vi "公式复合写入.vi"(11 "公式":cluster{"X^2":dbl, "X":dbl, "b":dbl}) -> ()   [LabVIEW 2016, in "斯坦道总磷.lvlib"]
uses:
  <vilib>/Utility/miscctls.llb/LVPointTypeDef.ctl
panel:
  out "连接的字符串":string
  in  "参数下拉列表":enum16{"总磷", "总氮"}(ring)
  in  "量程下拉列表":enum16{"低量程", "高量程"}(ring)
  in  "取消":bool
  in  "确认":bool
  in  "加标回收":bool
  in  "标样核查":bool
  in  "跨度核查":bool
  in  "空白核查":bool
  in  "水样测量":bool=TRUE
  # "请选择要写入的参数"
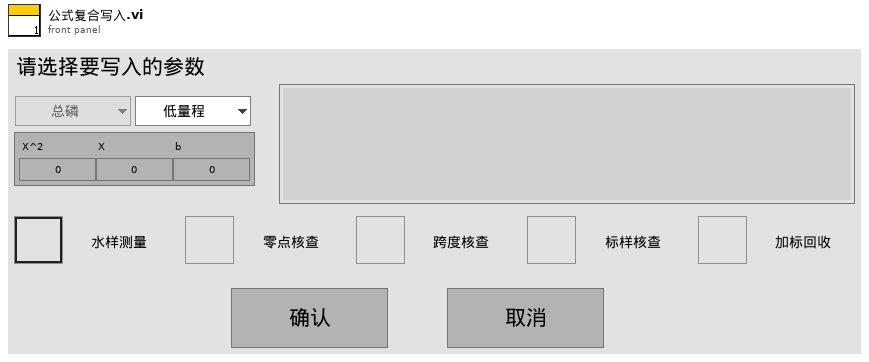
[diagram p1: front panel]
types:
  T1 = typedef "LVPointTypeDef.ctl" = cluster{"Horizontal":i16, "Vertical":i16}
  T2 = cluster{"测量量程":dbl, "测量精度":dbl, "测量间隔":dbl, "消解温度":dbl, "消解时长":dbl, "空白校准时间":timestamp, "曲线截距":dbl, "曲线斜率":dbl, "测量检出限":dbl, "测量信号值":dbl, "线性相关系数":dbl, "二次多项式系数":dbl, "标样校准时间":timestamp, "稀释倍数":dbl, "三项式系数":dbl, "空白标定系数":dbl, "量程系数":dbl, "F0/ORPA":dbl, "F1/ORPB":dbl, "F2/ORPK":dbl, "F3":dbl, "F4":dbl, "F5":dbl, "F6":dbl, "F7":dbl, "X0/滴定数":dbl, "量程":dbl}
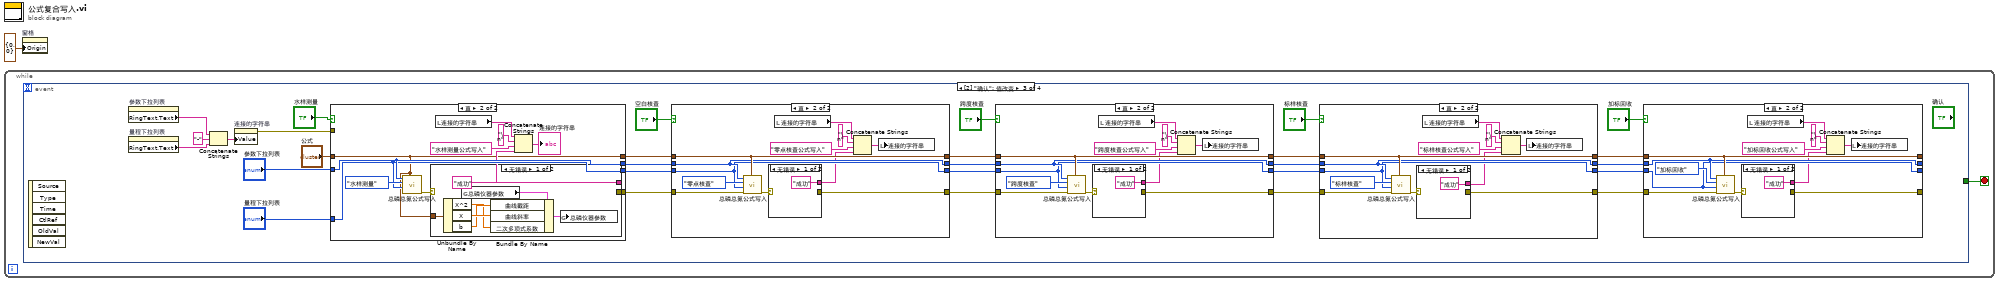
[diagram p0: block diagram]
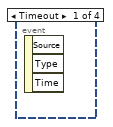
[diagram p2: hidden frame]
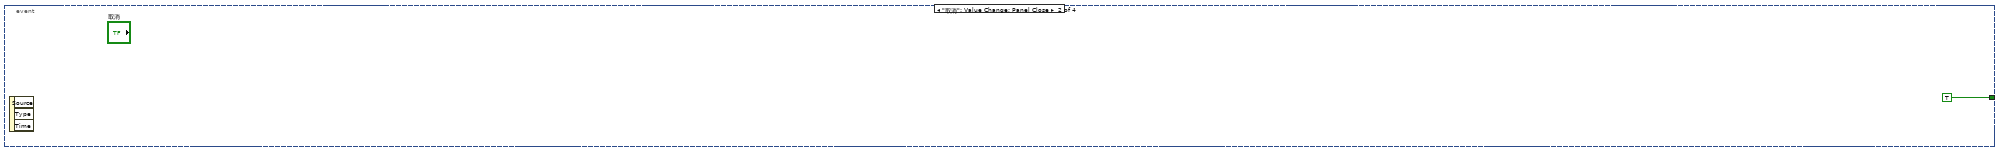
[diagram p3: hidden frame]
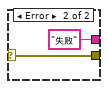
[diagram p5: hidden frame]
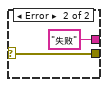
[diagram p7: hidden frame]
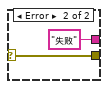
[diagram p9: hidden frame]
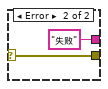
[diagram p11: hidden frame]
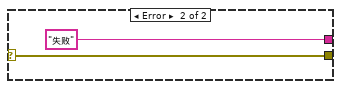
[diagram p13: hidden frame]
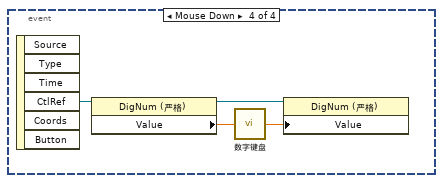
[diagram p14: hidden frame]
diagram:
  n1 = while {
    stop <- w2 stop-if-true
    n2 = event shown="[2] \"确认\": 值改变" {
      selector: _ -> [_ _ _ _]
      dyn-events: _ -> [_ _ _ _]
      timeout: _ -> [_ _ _ _]
      tunnel: [_ TRUE _ _] -> w2
      event Timeout {
        n3 = event-data() -> ()  [unwired: 1 in, 3 out]
      }
      event "取消": Value Change; Panel Close {
        n4 = event-data() -> ()  [unwired: 1 in, 3 out]
      }
      event "确认": Value Change {
        n5 = event-data() -> ()  [unwired: 1 in, 6 out]
        n6 = property on="参数下拉列表" class="Enum (严格)"() -> ("RingText.Text"=w6:string)  [unwired: 2 in, 2 out]
        n7 = property on="量程下拉列表" class="Enum (严格)"() -> ("RingText.Text"=w5:string)  [unwired: 2 in, 2 out]
        n8 = Concatenate Strings(w6, "-" ("字符串"), w5) -> (w7:string)
        n9 = property on="连接的字符串" class="Str"("Value"=w7) -> (error out=w8:errorcluster)  [unwired: 2 in, 1 out]
        n10 = case shown="真" "水样测量" {
          tunnel: "公式" -> [w107 w108]
          tunnel: "参数下拉列表" -> [w106 w117]
          tunnel: "量程下拉列表" -> [w105 w116]
          tunnel: [w107 w108] -> w28
          tunnel: [w106 w117] -> w27
          tunnel: [w105 w116] -> w26
          tunnel: [_ w114] -> w10
          tunnel: w8 -> [_ _]
          frame False {
          }
          frame True {
            n11 = call "总磷总氮公式写入.vi"("公式"=w108, "量程"=w116, "测量模式"=enum16{"水样测量", "零点核查", "跨度核查", "标样核查", "加标回收"}."水样测量", "测量参数"=w117) -> ("error out"=w115:errorcluster)  [unwired: 7 in]
            n12 = case shown="无错误" w115 {
              selector: w115 -> [_ w127]
              tunnel: [_ w127] -> w114
              tunnel: ["成功" "失败"] -> w113
              tunnel: w108 -> [w119 _]
              frame No Error {
                n13 = Unbundle By Name(w119) -> ("X^2"=w122:dbl, "X"=w124:dbl, "b"=w123:dbl)
                n14 = global read "总磷断电保存全局变量.vi" "总磷仪器参数"() -> (w121:T2)
                n15 = Bundle By Name(cluster=w121, "曲线截距"=w123, "曲线斜率"=w124, "二次多项式系数"=w122) -> (w120:T2)
                n16 = global write "总磷断电保存全局变量.vi" "总磷仪器参数"(w120) -> ()
              }
              frame Error {
              }
            }
            n17 = local read "连接的字符串"() -> (w110:string)
            n18 = Concatenate Strings(w110, "\n" ("字符串"), "水样测量公式写入", w113) -> (→"连接的字符串":string)
          }
        }
        n19 = case shown="真" "空白核查" {
          tunnel: w28 -> [w89 w100]
          tunnel: w27 -> [w88 w99]
          tunnel: w26 -> [w87 w98]
          tunnel: [_ w93] -> w25
          tunnel: [w89 w100] -> w24
          tunnel: [w88 w99] -> w23
          tunnel: [w87 w98] -> w22
          tunnel: w10 -> [_ w97]
          frame False {
          }
          frame True {
            n20 = call "总磷总氮公式写入.vi"("公式"=w100, "error in (no error)"=w97, "量程"=w98, "测量模式"=enum16{"水样测量", "零点核查", "跨度核查", "标样核查", "加标回收"}."零点核查", "测量参数"=w99) -> ("error out"=w94:errorcluster)  [unwired: 6 in]
            n21 = case shown="无错误" w94 {
              selector: w94 -> [_ w104]
              tunnel: [_ w104] -> w93
              tunnel: ["成功" "失败"] -> w95
              frame No Error {
              }
              frame Error {
              }
            }
            n22 = local read "连接的字符串"() -> (w92:string)
            n23 = Concatenate Strings(w92, "\n" ("字符串"), "零点核查公式写入", w95) -> (w90:string)
            n24 = local write "连接的字符串"(w90) -> ()
          }
        }
        n25 = case shown="真" "跨度核查" {
          tunnel: w24 -> [w71 w82]
          tunnel: w23 -> [w70 w81]
          tunnel: w22 -> [w69 w80]
          tunnel: [w71 w82] -> w21
          tunnel: [w70 w81] -> w19
          tunnel: [w69 w80] -> w18
          tunnel: w25 -> [_ w79]
          tunnel: [_ w72] -> w9
          frame False {
          }
          frame True {
            n26 = call "总磷总氮公式写入.vi"("公式"=w82, "error in (no error)"=w79, "量程"=w80, "测量模式"=enum16{"水样测量", "零点核查", "跨度核查", "标样核查", "加标回收"}."跨度核查", "测量参数"=w81) -> ("error out"=w73:errorcluster)  [unwired: 6 in]
            n27 = case shown="无错误" w73 {
              selector: w73 -> [_ w86]
              tunnel: [_ w86] -> w72
              tunnel: ["成功" "失败"] -> w74
              frame No Error {
              }
              frame Error {
              }
            }
            n28 = local read "连接的字符串"() -> (w76:string)
            n29 = Concatenate Strings(w76, "\n" ("字符串"), "跨度核查公式写入", w74) -> (w78:string)
            n30 = local write "连接的字符串"(w78) -> ()
          }
        }
        n31 = case shown="真" "标样核查" {
          tunnel: w21 -> [w53 w64]
          tunnel: w19 -> [w52 w63]
          tunnel: w18 -> [w51 w62]
          tunnel: [_ w54] -> w15
          tunnel: [w53 w64] -> w20
          tunnel: [w52 w63] -> w17
          tunnel: [w51 w62] -> w16
          tunnel: w9 -> [_ w61]
          frame False {
          }
          frame True {
            n32 = call "总磷总氮公式写入.vi"("公式"=w64, "error in (no error)"=w61, "量程"=w62, "测量模式"=enum16{"水样测量", "零点核查", "跨度核查", "标样核查", "加标回收"}."标样核查", "测量参数"=w63) -> ("error out"=w55:errorcluster)  [unwired: 6 in]
            n33 = case shown="无错误" w55 {
              selector: w55 -> [_ w68]
              tunnel: [_ w68] -> w54
              tunnel: ["成功" "失败"] -> w56
              frame No Error {
              }
              frame Error {
              }
            }
            n34 = local read "连接的字符串"() -> (w58:string)
            n35 = Concatenate Strings(w58, "\n" ("字符串"), "标样核查公式写入", w56) -> (w60:string)
            n36 = local write "连接的字符串"(w60) -> ()
          }
        }
        n37 = case shown="真" "加标回收" {
          tunnel: w20 -> [w35 w46]
          tunnel: w17 -> [w34 w45]
          tunnel: w16 -> [w33 w44]
          tunnel: [w35 w46] -> _
          tunnel: [w34 w45] -> _
          tunnel: [w33 w44] -> _
          tunnel: w15 -> [_ w43]
          tunnel: [_ w36] -> _
          frame False {
          }
          frame True {
            n38 = call "总磷总氮公式写入.vi"("公式"=w46, "error in (no error)"=w43, "量程"=w44, "测量模式"=enum16{"水样测量", "零点核查", "跨度核查", "标样核查", "加标回收"}."加标回收", "测量参数"=w45) -> ("error out"=w37:errorcluster)  [unwired: 6 in]
            n39 = case shown="无错误" w37 {
              selector: w37 -> [_ w50]
              tunnel: [_ w50] -> w36
              tunnel: ["成功" "失败"] -> w38
              frame No Error {
              }
              frame Error {
              }
            }
            n40 = local read "连接的字符串"() -> (w40:string)
            n41 = Concatenate Strings(w40, "\n" ("字符串"), "加标回收公式写入", w38) -> (w42:string)
            n42 = local write "连接的字符串"(w42) -> ()
          }
        }
      }
      event "公式.X^2", "公式.X", "公式.b": Mouse Down {
        n43 = event-data() -> ("CtlRef"=w131:refnum<vi>)  [unwired: 1 in, 5 out]
        n44 = property class="DigNum (严格)"(reference=w131) -> (reference out=w128:refnum<vi>, "Value"=w130:dbl)  [unwired: 1 in, 1 out]
        n45 = call "数字键盘.vi"("OldNumber"=w130) -> ("NewNumber"=w129:dbl)
        n46 = property class="DigNum (严格)"(reference=w128, "Value"=w129) -> ()  [unwired: 1 in, 2 out]
      }
    }
  }
  n47 = property on="窗格" class="Pane"("Origin"=T1 {"Horizontal"=0, "Vertical"=0} ("原点")) -> ()  [unwired: 2 in, 2 out]
